vi "Key Codes Constants.vi"() -> ()   [LabVIEW 2021, in "Seq Edit Quick Drop.lvlib"]
uses:
  Seq Edit Quick Drop.lvlib
  Key Codes Constants.ctl
panel:
  in  "Key Codes Constants":T1=[{"Code"=48, "Key"="0"}, {"Code"=49, "Key"="1"}, {"Code"=50, "Key"="2"}, {"Code"=51, "Key"="3"}, {"Code"=52, "Key"="4"}, {"Code"=53, "Key"="5"}, {"Code"=54, "Key"="6"}, {"Code"=55, "Key"="7"}, {"Code"=56, "Key"="8"}, {"Code"=57, "Key"="9"}, {"Code"=65, "Key"="A"}, {"Code"=30, "Key"="ACCEPT"}, {"Code"=107, "Key"="ADD"}, {"Code"=93, "Key"="APPS"}, {"Code"=66, "Key"="B"}, {"Code"=8, "Key"="BACK"}, {"Code"=67, "Key"="C"}, {"Code"=3, "Key"="CANCEL"}, {"Code"=20, "Key"="CAPITAL"}, {"Code"=12, "Key"="CLEAR"}, {"Code"=17, "Key"="CONTROL"}, {"Code"=28, "Key"="CONVERT"}, {"Code"=68, "Key"="D"}, {"Code"=110, "Key"="DECIMAL"}, {"Code"=46, "Key"="DELETE"}, {"Code"=111, "Key"="DIVIDE"}, {"Code"=40, "Key"="DOWN"}, {"Code"=69, "Key"="E"}, {"Code"=35, "Key"="END"}, {"Code"=27, "Key"="ESCAPE"}, {"Code"=43, "Key"="EXECUTE"}, {"Code"=70, "Key"="F"}, {"Code"=112, "Key"="F1"}, {"Code"=121, "Key"="F10"}, {"Code"=122, "Key"="F11"}, {"Code"=123, "Key"="F12"}, {"Code"=124, "Key"="F13"}, {"Code"=125, "Key"="F14"}, {"Code"=126, "Key"="F15"}, {"Code"=127, "Key"="F16"}, {"Code"=128, "Key"="F17"}, {"Code"=129, "Key"="F18"}, {"Code"=130, "Key"="F19"}, {"Code"=113, "Key"="F2"}, {"Code"=131, "Key"="F20"}, {"Code"=132, "Key"="F21"}, {"Code"=133, "Key"="F22"}, {"Code"=134, "Key"="F23"}, {"Code"=135, "Key"="F24"}, {"Code"=114, "Key"="F3"}, {"Code"=115, "Key"="F4"}, {"Code"=116, "Key"="F5"}, {"Code"=117, "Key"="F6"}, {"Code"=118, "Key"="F7"}, {"Code"=119, "Key"="F8"}, {"Code"=120, "Key"="F9"}, {"Code"=24, "Key"="FINAL"}, {"Code"=71, "Key"="G"}, {"Code"=72, "Key"="H"}, {"Code"=21, "Key"="HANGEUL"}, {"Code"=21, "Key"="HANGUL"}, {"Code"=25, "Key"="HANJA"}, {"Code"=47, "Key"="HELP"}, {"Code"=36, "Key"="HOME"}, {"Code"=73, "Key"="I"}, {"Code"=45, "Key"="INSERT"}, {"Code"=74, "Key"="J"}, {"Code"=23, "Key"="JUNJA"}, {"Code"=75, "Key"="K"}, {"Code"=21, "Key"="KANA"}, {"Code"=25, "Key"="KANJI"}, {"Code"=76, "Key"="L"}, {"Code"=37, "Key"="LEFT"}, {"Code"=91, "Key"="LWIN"}, {"Code"=77, "Key"="M"}, {"Code"=18, "Key"="ALT"}, {"Code"=31, "Key"="MODECHANGE"}, {"Code"=106, "Key"="MULTIPLY"}, {"Code"=78, "Key"="N"}, {"Code"=34, "Key"="NEXT"}, {"Code"=29, "Key"="NONCONVERT"}, {"Code"=144, "Key"="NUMLOCK"}, {"Code"=96, "Key"="NUMPAD0"}, {"Code"=97, "Key"="NUMPAD1"}, {"Code"=98, "Key"="NUMPAD2"}, {"Code"=99, "Key"="NUMPAD3"}, {"Code"=100, "Key"="NUMPAD4"}, {"Code"=101, "Key"="NUMPAD5"}, {"Code"=102, "Key"="NUMPAD6"}, {"Code"=103, "Key"="NUMPAD7"}, {"Code"=104, "Key"="NUMPAD8"}, {"Code"=105, "Key"="NUMPAD9"}, {"Code"=79, "Key"="O"}, {"Code"=80, "Key"="P"}, {"Code"=19, "Key"="PAUSE"}, {"Code"=42, "Key"="PRINT"}, {"Code"=33, "Key"="PRIOR"}, {"Code"=81, "Key"="Q"}, {"Code"=82, "Key"="R"}, {"Code"=13, "Key"="RETURN"}, {"Code"=39, "Key"="RIGHT"}, {"Code"=92, "Key"="RWIN"}, {"Code"=83, "Key"="S"}, {"Code"=145, "Key"="SCROLL"}, {"Code"=41, "Key"="SELECT"}, {"Code"=108, "Key"="SEPARATOR"}, {"Code"=16, "Key"="SHIFT"}, {"Code"=44, "Key"="SNAPSHOT"}, {"Code"=32, "Key"="SPACE"}, {"Code"=109, "Key"="SUBTRACT"}, {"Code"=84, "Key"="T"}, {"Code"=9, "Key"="TAB"}, {"Code"=85, "Key"="U"}, {"Code"=38, "Key"="UP"}, {"Code"=86, "Key"="V"}, {"Code"=87, "Key"="W"}, {"Code"=88, "Key"="X"}, {"Code"=89, "Key"="Y"}, {"Code"=90, "Key"="Z"}] {"Code" format="%02x"}
  # "These constants specify the virtual key codes for the KeyDown and KeyUp events in TestStand. \n\nhttps://zone.ni.com/reference/en-XX/help/370052AA-01/tsuiref/reftopics/keycodes/"
  # "DO NOT MODIFY"
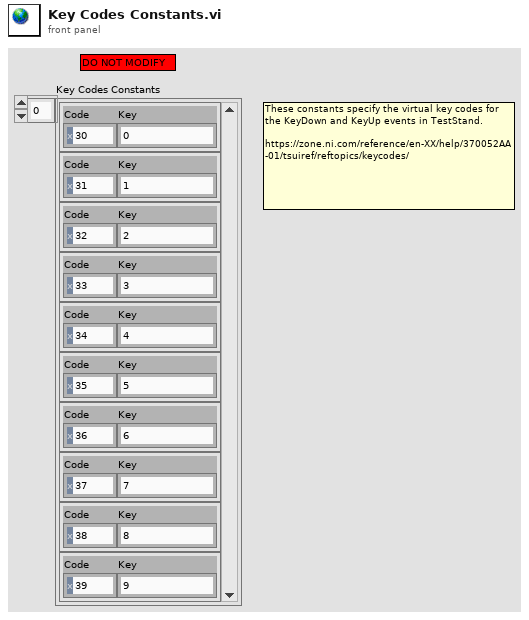
[diagram p1: front panel]
types:
  T1 = typedef "Seq Edit Quick Drop.lvlib/Key Codes Constants.ctl" = cluster{"Code":i16, "Key":string}[]
diagram:
